vi "UsrProfiles-Format for last profiles used.vi"() -> (0 "error out":errorcluster, 1 "Selected profile name":string, 2 "Key setup":T1)   [LabVIEW 2013]
uses:
  Globals/gl_UsrProfiles globals.vi
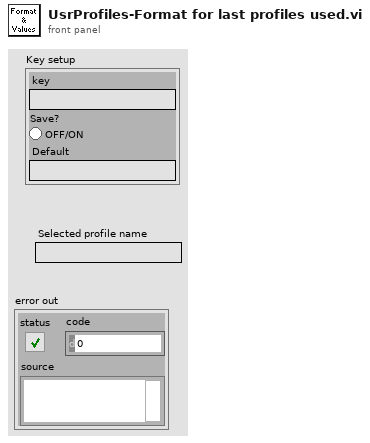
[diagram p1: front panel]
types:
  T1 = cluster{"key":string, "Save?":bool, "Default":string}
  T2 = typedef "User login window refs.ctl" = cluster{"User profiles window ref":refnum<k9>, "Users listbox":refnum<vi>, "Profiles listbox":refnum<vi>, "Last used":refnum<vi>}
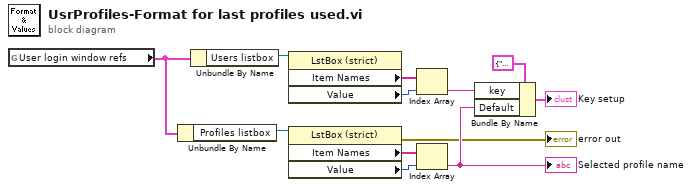
[diagram p0: block diagram]
diagram:
  n1 = global read "gl_UsrProfiles globals.vi" "User login window refs"() -> (w1:T2)
  n2 = Unbundle By Name(w1) -> ("Profiles listbox"=w6:refnum<vi>)
  n3 = Unbundle By Name(w1) -> ("Users listbox"=w12:refnum<vi>)
  n4 = property class="LstBox (strict)"(reference=w12) -> ("Item Names"=w11:string[], "Value"=w10:i32)  [unwired: 1 in, 2 out]
  n5 = property class="LstBox (strict)"(reference=w6) -> (error out=→"error out":errorcluster, "Item Names"=w5:string[], "Value"=w4:i32)  [unwired: 1 in, 1 out]
  n6 = Index Array(array=w11, index=w10) -> (element=w8:string)
  n7 = Index Array(array=w5, index=w4) -> (element=w3:string)
  "Selected profile name" <- w3
  n8 = Bundle By Name(cluster=T1 {"key"="", "Save?"=TRUE, "Default"=""}, "key"=w8, "Default"=w3) -> (→"Key setup":T1)
